vi "subInitializeFor5Choice.vi"(0 "Arduino Resource":T1={"VISA resource"="", "Board Type"=enum."Uno", "Connection Type"=enum."USB / Serial", "Bytes Per Packet (15)"=15}, 5 "LED Start Pin":i32, 7 "Detector Start Pin":i32, 11 "error in":errorcluster) -> (4 "Arduino Resource 2":T1={"VISA resource"="", "Board Type"=enum."Uno", "Connection Type"=enum."USB / Serial", "Bytes Per Packet (15)"=15}, 15 "error out":errorcluster)   [LabVIEW 2016]
uses:
  <vilib>/LabVIEW Interface for Arduino/Type Defs/Arduino Resource.ctl
  <vilib>/LabVIEW Interface for Arduino/Type Defs/Board Type.ctl
  <vilib>/LabVIEW Interface for Arduino/Type Defs/Pin Mode.ctl
  <vilib>/LabVIEW Interface for Arduino/LabVIEW Interface for Arduino.lvlib
panel:
  # "FIXED : \nStepper Motor Pin : 2,3,4,5\nPellet Box : 9\nHouse Light : 8"
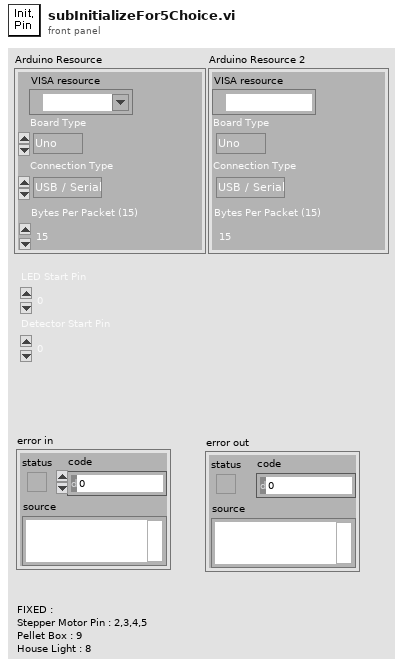
[diagram p1: front panel]
types:
  T1 = typedef "LabVIEW Interface for Arduino.lvlib/Arduino Resource.ctl" = cluster{"VISA resource":refnum<visa-resource-name>, "Board Type":T2, "Connection Type":enum8{"USB / Serial"}, "Bytes Per Packet (15)":u8}
  T2 = typedef "LabVIEW Interface for Arduino.lvlib/Board Type.ctl" = enum16{"Uno", "Dimuelanove w/Atmega 328", "Mega 2560"}
  T3 = typedef "LabVIEW Interface for Arduino.lvlib/Pin Mode.ctl" = enum8{"Input", "Output"}
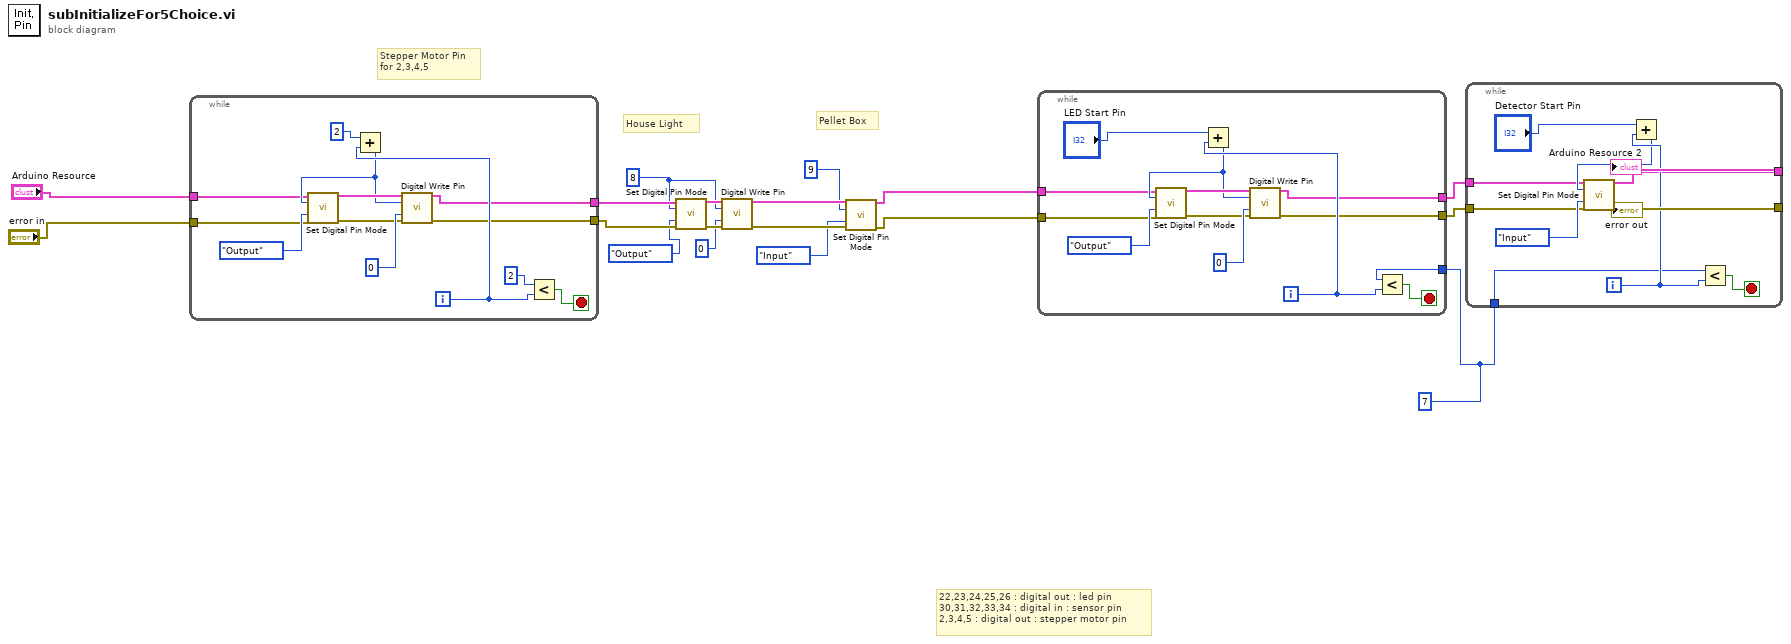
[diagram p0: block diagram]
diagram:
  w4 = 8
  w14 = 7
  # "Pellet Box"
  # "House Light"
  # "Stepper Motor Pin\nfor 2,3,4,5"
  # "22,23,24,25,26 : digital out : led pin\n30,31,32,33,34 : digital in : sensor pin\n2,3,4,5 : digital out : stepper motor pin"
  n1 = while {
    tunnel: [w24] -> w13
    tunnel: [w23] -> w9
    tunnel: "Arduino Resource" -> [w22]
    tunnel: "error in" -> [w21]
    i -> [w30]
    stop <- w32 stop-if-true
    n2 = Add(x=2, y=w30) -> (x+y=w26:i32)
    n3 = call <vilib>:"Set Digital Pin Mode.vi"("Arduino Resource"=w22, "Digital I/O Pin"=w26, "Pin Mode (Input)"=Pin_Mode."Output", "error in"=w21) -> ("Arduino Resource"=w28:T1, "error out"=w27:errorcluster)  [unwired: 10 in]
    n4 = call <vilib>:"Digital Write Pin.vi"("Arduino Resource"=w28, "Digital I/O Pin (0)"=w26, "Value (0)"=0, "error in"=w27) -> ("Arduino Resource"=w24:T1, "error out"=w23:errorcluster)  [unwired: 10 in]
    n5 = Less?(x=2, y=w30) -> (x < y?=w32:bool)
  }
  n6 = call <vilib>:"Set Digital Pin Mode.vi"("Arduino Resource"=w13, "Digital I/O Pin"=w4, "Pin Mode (Input)"=Pin_Mode."Output", "error in"=w9) -> ("Arduino Resource"=w12:T1, "error out"=w8:errorcluster)  [unwired: 10 in]
  n7 = call <vilib>:"Digital Write Pin.vi"("Arduino Resource"=w12, "Digital I/O Pin (0)"=w4, "Value (0)"=0, "error in"=w8) -> ("Arduino Resource"=w11:T1, "error out"=w7:errorcluster)  [unwired: 10 in]
  n8 = call <vilib>:"Set Digital Pin Mode.vi"("Arduino Resource"=w11, "Digital I/O Pin"=9, "Pin Mode (Input)"=Pin_Mode."Input", "error in"=w7) -> ("Arduino Resource"=w10:T1, "error out"=w6:errorcluster)  [unwired: 10 in]
  n9 = while {
    tunnel: [w39] -> w20
    tunnel: [w38] -> w19
    tunnel: w10 -> [w37]
    tunnel: w6 -> [w36]
    tunnel: w14 -> [w34]
    i -> [w44]
    stop <- w45 stop-if-true
    n10 = Add(x="LED Start Pin", y=w44) -> (x+y=w41:i32)
    n11 = call <vilib>:"Set Digital Pin Mode.vi"("Arduino Resource"=w37, "Digital I/O Pin"=w41, "Pin Mode (Input)"=Pin_Mode."Output", "error in"=w36) -> ("Arduino Resource"=w43:T1, "error out"=w42:errorcluster)  [unwired: 10 in]
    n12 = call <vilib>:"Digital Write Pin.vi"("Arduino Resource"=w43, "Digital I/O Pin (0)"=w41, "Value (0)"=0, "error in"=w42) -> ("Arduino Resource"=w39:T1, "error out"=w38:errorcluster)  [unwired: 10 in]
    n13 = Less?(x=w34, y=w44) -> (x < y?=w45:bool)
  }
  n14 = while {
    tunnel: w20 -> [w52]
    tunnel: w19 -> [w51]
    tunnel: [w50] -> w17
    tunnel: [w49] -> w18
    tunnel: w14 -> [w47]
    i -> [w55]
    stop <- w56 stop-if-true
    n15 = Add(x="Detector Start Pin", y=w55) -> (x+y=w54:i32)
    n16 = call <vilib>:"Set Digital Pin Mode.vi"("Arduino Resource"=w52, "Digital I/O Pin"=w54, "Pin Mode (Input)"=Pin_Mode."Input", "error in"=w51) -> ("Arduino Resource"=w50:T1, "error out"=w49:errorcluster)  [unwired: 10 in]
    n17 = Less?(x=w47, y=w55) -> (x < y?=w56:bool)
  }
  "Arduino Resource 2" <- w17
  "error out" <- w18
